vi "YPR_SubVI_string.vi"(8 "error in":errorcluster, 11 "read buffer":string) -> (0 "error out":errorcluster, 1 "Roll":sgl format="%#_10g", 2 "Pitch":sgl format="%#_10g", 3 "Yaw":sgl format="%#_10g")   [LabVIEW 2016]
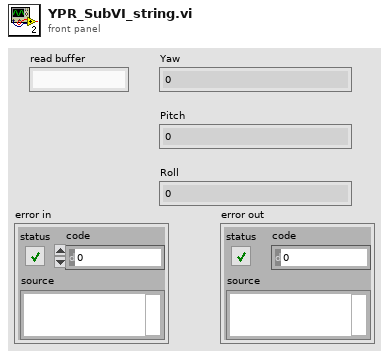
[diagram p1: front panel]
types:
  T1 = enum16{"big-endian, network order", "native, host order", "little-endian"}
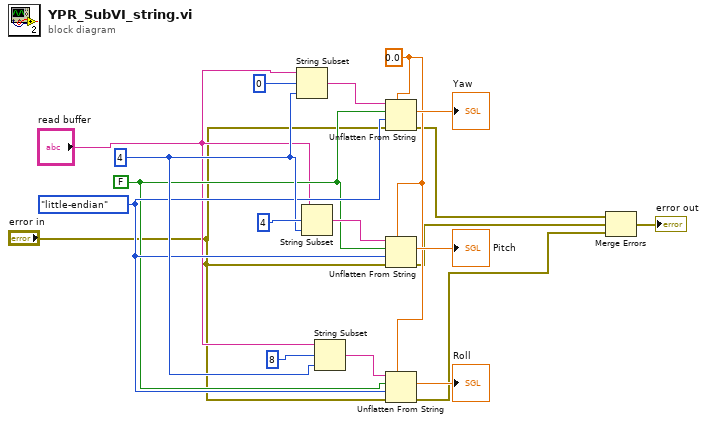
[diagram p0: block diagram]
diagram:
  w7 = sgl 0.0
  w8 = FALSE ("data includes array or string size? (T)")
  w9 = T1."little-endian" ("byte order (0:big-endian, network order)")
  w10 = 4
  n1 = String Subset(string="read buffer", offset (0)=0, length (rest)=w10) -> (substring=w13:string)
  n2 = String Subset(string="read buffer", offset (0)=4, length (rest)=w10) -> (substring=w16:string)
  n3 = String Subset(string="read buffer", offset (0)=8, length (rest)=w10) -> (substring=w19:string)
  n4 = Unflatten From String(type=w7, binary string=w13, data includes array or string size? (T)=w8, byte order (0:big-endian, network order)=w9, error in (no error)="error in") -> (value=→"Yaw":sgl, error out=w4:errorcluster)  [unwired: 1 out]
  n5 = Unflatten From String(type=w7, binary string=w16, data includes array or string size? (T)=w8, byte order (0:big-endian, network order)=w9, error in (no error)="error in") -> (value=→"Pitch":sgl, error out=w3:errorcluster)  [unwired: 1 out]
  n6 = Unflatten From String(type=w7, binary string=w19, data includes array or string size? (T)=w8, byte order (0:big-endian, network order)=w9, error in (no error)="error in") -> (value=→"Roll":sgl, error out=w2:errorcluster)  [unwired: 1 out]
  n7 = Merge Errors(w4, w3, w2) -> (→"error out":errorcluster)
